vi "Read position.vi"(8 "error in (no error)":errorcluster, 11 "VISA Refnum in":refnum<visa-resource-name>) -> (0 "error out":errorcluster, 2 "End position?":bool, 3 "Position":i32)   [LabVIEW 2020, in "Arduino stepper.lvlib"]
uses:
  Arduino stepper.lvlib
  <vilib>/Instr/_visa.llb/VISA Flush IO Buffer Mask.ctl
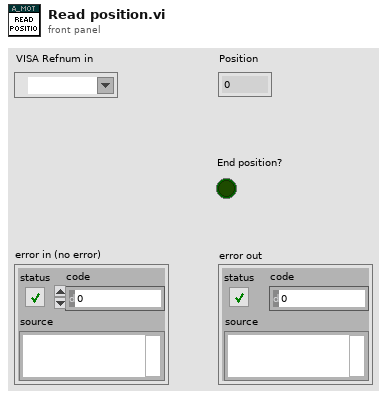
[diagram p1: front panel]
types:
  T1 = typedef "VISA Flush IO Buffer Mask.ctl" = u16
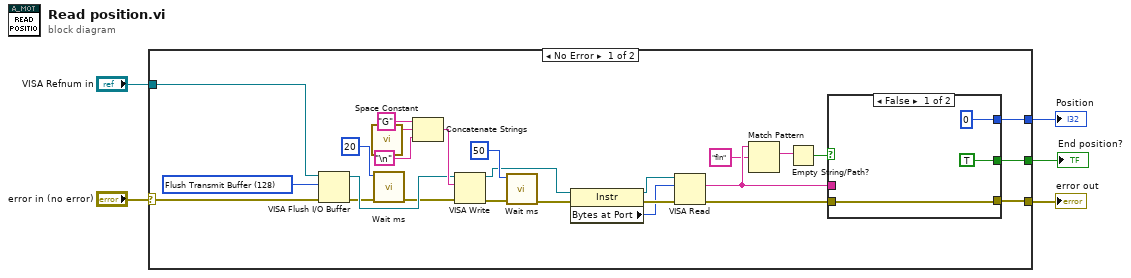
[diagram p0: block diagram]
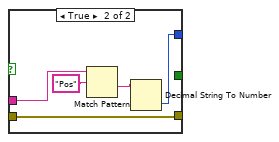
[diagram p2: hidden frame]
diagram:
  n1 = case shown="No Error" "error in (no error)" {
    selector: "error in (no error)" -> [w21 w40]
    tunnel: [w12 w40] -> w5
    tunnel: "VISA Refnum in" -> [w23 _]
    tunnel: [w20 _] -> w2
    tunnel: [w7 _] -> w1
    frame No Error {
      w14 = T1 128 items=["Flush Receive Buffer"=16, "Write Transmit Buffer to Device"=32, "Flush Receive Buffer (No I/O)"=64, "Flush Transmit Buffer"=128] ("Mask")
      n2 = VISA Flush I/O Buffer(VISA resource name=w23, mask (16)=w14, error in (no error)=w21) -> (VISA resource name out=w28:refnum<visa-resource-name>, error out=w22:errorcluster)
      n3 = call <vilib>:"Space Constant.vi"() -> ("String"=w6:string)
      n4 = call "Wait ms.vi"("error in (no error)"=w22, "milliseconds to wait"=u32 20) -> ("error out"=w27:errorcluster)  [unwired: 9 in]
      n5 = Concatenate Strings("G" ("string"), w6, "\n") -> (w29:string)
      n6 = VISA Write(VISA resource name=w28, write buffer=w29, error in (no error)=w27) -> (VISA resource name out=w17:refnum<visa-resource-name>, error out=w30:errorcluster)  [unwired: 1 out]
      n7 = call "Wait ms.vi"("error in (no error)"=w30, "milliseconds to wait"=u32 50) -> ("error out"=w19:errorcluster)  [unwired: 9 in]
      n8 = property class="Instr"(reference=w17, error in=w19) -> (reference out=w16:refnum<visa-resource-name>, error out=w18:errorcluster, "Bytes at Port"=w15:u32)
      n9 = VISA Read(VISA resource name=w16, byte count=w15, error in (no error)=w18) -> (read buffer=w11:string, error out=w13:errorcluster)  [unwired: 2 out]
      n10 = Match Pattern(string=w11, regular expression="fin") -> (match substring=w9:string)  [unwired: 1 in, 3 out]
      n11 = Empty String/Path?(string/path=w9) -> (empty?=w8:bool)
      n12 = case shown="False" w8 {
        tunnel: w11 -> [_ w39]
        tunnel: [0 w36] -> w20
        tunnel: w13 -> [w34 w35]
        tunnel: [w34 w35] -> w12
        tunnel: [TRUE _] -> w7
        frame False {
        }
        frame True {
          n13 = Match Pattern(string=w39, regular expression="Pos") -> (after substring=w37:string)  [unwired: 1 in, 3 out]
          n14 = Decimal String To Number(string=w37) -> (number=w36:i32)  [unwired: 2 in, 1 out]
        }
      }
    }
    frame Error {
    }
  }
  "error out" <- w5
  "Position" <- w2
  "End position?" <- w1
